vi "Parse Serial Response.vi"(7 "Response Syntax":T1, 8 "error in (no error)":errorcluster, 10 "Raw Response":string) -> (0 "error out":errorcluster, 1 "Parsed Double":dbl, 2 "Parsed String":string, 4 "As expected?":bool)   [LabVIEW 2017, in "Drivers.lvlib" / "ASI TG-1000.lvlib"]
uses:
  ASI TG-1000.lvlib
  Serial Response Syntax.ctl
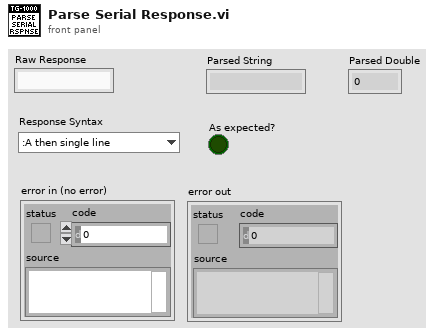
[diagram p1: front panel]
types:
  T1 = typedef "Drivers.lvlib/ASI TG-1000.lvlib/Serial Response Syntax.ctl" = enum16{":A then single line", "Single line, no :A", ":A or : then single line", ":A then single number", ":A or : then single number", ":A then <axis>= single number"}
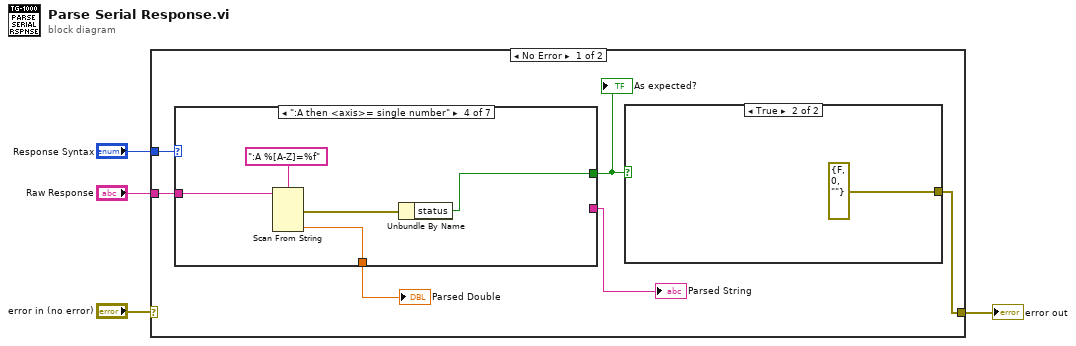
[diagram p0: block diagram]
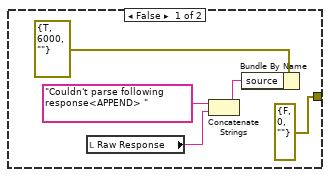
[diagram p2: hidden frame]
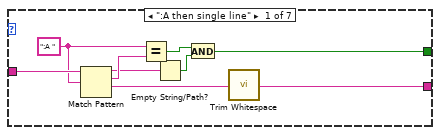
[diagram p3: hidden frame]
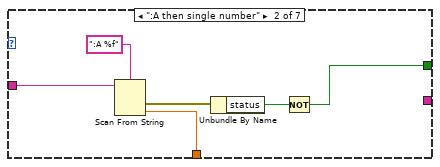
[diagram p4: hidden frame]
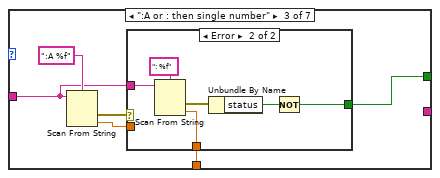
[diagram p5: hidden frame]
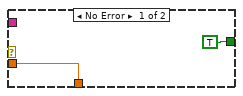
[diagram p6: hidden frame]
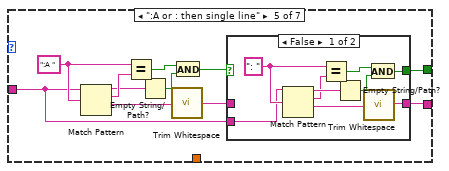
[diagram p7: hidden frame]
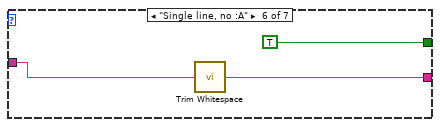
[diagram p9: hidden frame]
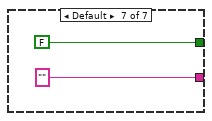
[diagram p10: hidden frame]
diagram:
  n1 = case shown="No Error" "error in (no error)" {
    selector: "error in (no error)" -> [_ w78]
    tunnel: "Response Syntax" -> [w10 _]
    tunnel: "Raw Response" -> [w9 _]
    tunnel: [w6 w78] -> w1
    frame No Error {
      n2 = case shown="\":A then <axis>= single number\"" w10 {
        tunnel: w9 -> [w25 w30 w32 w50 w51 w74 _]
        tunnel: [w18 _ _ _ w52 w73 "" ("Raw Response")] -> w8
        tunnel: [w19 w26 w33 w46 w54 TRUE FALSE] -> w7
        tunnel: [_ w29 w35 w48 _ _ _] -> w5
        frame ":A then single line" {
          w23 = ":A " ("regular expression")
          n3 = Match Pattern(string=w25, regular expression=w23) -> (before substring=w22:string, match substring=w24:string, after substring=w17:string)  [unwired: 1 in, 1 out]
          n4 = Equal?(x=w23, y=w24) -> (x = y?=w21:bool)
          n5 = Empty String/Path?(string/path=w22) -> (empty?=w20:bool)
          n6 = And(x=w21, y=w20) -> (x .and. y?=w19:bool)
          n7 = call <vilib>:"Trim Whitespace.vi"("string"=w17) -> ("trimmed string"=w18:string)  [unwired: 1 in]
        }
        frame ":A then single number" {
          n8 = Scan From String(format string=":A %f" ("regular expression"), input string=w30) -> (error out=w28:errorcluster, output 1=w29:dbl)  [unwired: 3 in, 2 out]
          n9 = Unbundle By Name(w28) -> ("status"=w27:bool)
          n10 = Not(x=w27) -> (.not. x?=w26:bool)
        }
        frame ":A or : then single number" {
          n11 = Scan From String(format string=":A %f" ("regular expression"), input string=w32) -> (error out=w36:errorcluster, output 1=w34:dbl)  [unwired: 3 in, 2 out]
          n12 = case shown="Error" w36 {
            tunnel: [w39 w44] -> w35
            tunnel: w34 -> [w39 _]
            tunnel: [TRUE w42] -> w33
            tunnel: w32 -> [_ w41]
            frame No Error {
            }
            frame Error {
              n13 = Scan From String(format string=": %f" ("regular expression"), input string=w41) -> (error out=w43:errorcluster, output 1=w44:dbl)  [unwired: 3 in, 2 out]
              n14 = Unbundle By Name(w43) -> ("status"=w40:bool)
              n15 = Not(x=w40) -> (.not. x?=w42:bool)
            }
          }
        }
        frame ":A then <axis>= single number" {
          n16 = Scan From String(format string=":A %[A-Z]=%f" ("regular expression"), input string=w50) -> (error out=w47:errorcluster, output 2=w48:dbl)  [unwired: 5 in, 2 out]
          n17 = Unbundle By Name(w47) -> ("status"=w46:bool)
        }
        frame ":A or : then single line" {
          w60 = ":A " ("regular expression")
          n18 = Match Pattern(string=w51, regular expression=w60) -> (before substring=w59:string, match substring=w61:string, after substring=w56:string)  [unwired: 1 in, 1 out]
          n19 = Equal?(x=w60, y=w61) -> (x = y?=w58:bool)
          n20 = Empty String/Path?(string/path=w59) -> (empty?=w57:bool)
          n21 = call <vilib>:"Trim Whitespace.vi"("string"=w56) -> ("trimmed string"=w53:string)  [unwired: 1 in]
          n22 = And(x=w58, y=w57) -> (x .and. y?=w55:bool)
          n23 = case shown="False" w55 {
            selector: w55 -> [_ w72]
            tunnel: [w64 w72] -> w54
            tunnel: w53 -> [_ w71]
            tunnel: [w63 w71] -> w52
            tunnel: w51 -> [w62 _]
            frame False {
              w66 = ": " ("regular expression")
              n24 = Match Pattern(string=w62, regular expression=w66) -> (before substring=w67:string, match substring=w65:string, after substring=w70:string)  [unwired: 1 in, 1 out]
              n25 = Equal?(x=w66, y=w65) -> (x = y?=w68:bool)
              n26 = Empty String/Path?(string/path=w67) -> (empty?=w69:bool)
              n27 = call <vilib>:"Trim Whitespace.vi"("string"=w70) -> ("trimmed string"=w63:string)  [unwired: 1 in]
              n28 = And(x=w68, y=w69) -> (x .and. y?=w64:bool)
            }
            frame True {
            }
          }
        }
        frame "Single line, no :A" {
          n29 = call <vilib>:"Trim Whitespace.vi"("string"=w74) -> ("trimmed string"=w73:string)  [unwired: 1 in]
        }
        frame Default {
        }
      }
      "Parsed String" <- w8
      "As expected?" <- w7
      "Parsed Double" <- w5
      n30 = case shown="True" w7 {
        tunnel: [errorcluster {"status"=FALSE, "code"=0, "source"=""} ("error IO") errorcluster {"status"=FALSE, "code"=0, "source"=""} ("error IO")] -> w6
        frame False {
          n31 = local read "Raw Response"() -> (w12:string)
          n32 = Concatenate Strings("Couldn't parse following response<APPEND> " ("source"), w12) -> (w13:string)
          n33 = Bundle By Name(cluster=errorcluster {"status"=TRUE, "code"=6000, "source"=""} ("error IO"), "source"=w13) -> ()  [unwired: 1 out]
        }
        frame True {
        }
      }
    }
    frame Error {
    }
  }
  "error out" <- w1
